vi "test_ccd_timerResolution.vi"(8 "error in":errorcluster, 11 "CCD in":refnum<class "CCD.lvclass">) -> (0 "error out":errorcluster, 3 "CCD out":refnum<class "CCD.lvclass">)   [LabVIEW 2023, in "horiba.test.lvlib"]
uses:
  horiba.test.lvlib
  Classes/CCD/CCD.lvclass
  C:/Projects/Horiba/horiba-labview-sdk/Source/Classes/GenericDevice/GenericDevice.lvclass
  15e7fe39-3d4f-4ccc-ae5c-22e5f2c5c50b.vi
  <vilib>/addons/_JKI Toolkits/Caraya/classes/Assert/Assert Equal Value and Type_Variant.vi
  <vilib>/addons/_JKI Toolkits/Caraya/classes/Test/Test.lvclass
  <vilib>/addons/_JKI Toolkits/Caraya/classes/Assert/Assert.lvclass
  <userlib>/_OpenG.lib/lvdata/lvdata.llb/openg_variant.lvlib
panel:
  # "Connector Pane"
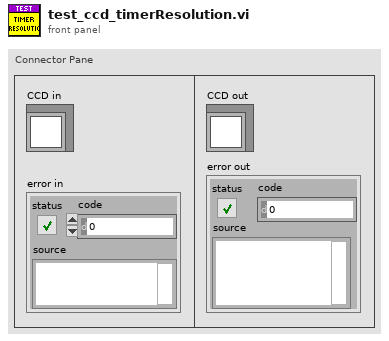
[diagram p1: front panel]
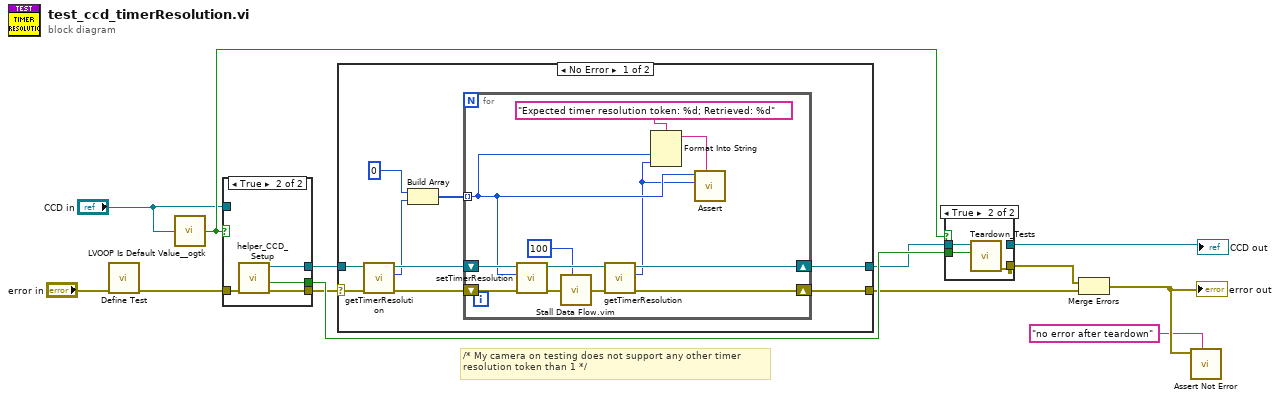
[diagram p0: block diagram]
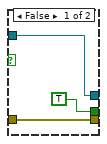
[diagram p3: hidden frame]
diagram:
  # "/* My camera on testing does not support any other timer \nresolution token than 1 */"
  n1 = call <vilib>:"Define Test.vi"("error in (no error)"="error in") -> ("error out"=w8:errorcluster)  [unwired: 9 in, 1 out]
  n2 = call <userlib>:"LVOOP Is Default Value__ogtk.vi"("Object"="CCD in") -> ("Is Default Value?"=w9:bool)
  n3 = case shown="True" w9 {
    tunnel: w8 -> [w15 w20]
    tunnel: [w15 w19] -> w4
    tunnel: [w16 w18] -> w6
    tunnel: [TRUE ("Module Was Already Running?") w17] -> w10
    tunnel: "CCD in" -> [w16 _]
    frame False {
    }
    frame True {
      n4 = call "helper_CCD_Setup.vi"("error in"=w20) -> ("error out"=w19:errorcluster, "Module Was Already Running?"=w17:bool, "CCD out"=w18:refnum<class "CCD.lvclass">)  [unwired: 7 in, 1 out]
    }
  }
  n5 = case shown="No Error" w4 {
    selector: w4 -> [w29 w42]
    tunnel: [w26 w43] -> w5
    tunnel: w6 -> [w28 w43]
    tunnel: [w24 w42] -> w3
    frame No Error {
      n6 = call "getTimerResolution.vi"("error in (no error)"=w29, "CCD in"=w28) -> ("error out"=w25:errorcluster, "resolutionToken"=w22:i32, "CCD out"=w27:refnum<class "CCD.lvclass">)  [unwired: 7 in]
      n7 = Build Array(0 ("token"), w22) -> (w21:i32[])
      n8 = for {
        shift-right: [w38] -> w26
        shift-left: w27 -> [w39]
        shift-right: [w36] -> w24
        shift-left: w25 -> [w37]
        tunnel: w21 -> [w33] mode=indexing
        n9 = call "setTimerResolution.vi"("error in (no error)"=w37, "resolutionToken"=w33, "CCD in"=w39) -> ("error out"=w41:errorcluster, "CCD out"=w40:refnum<class "CCD.lvclass">)  [unwired: 5 in, 2 out]
        n10 = call "Stall Data Flow.vim"("value in"=w41, "milliseconds to wait"=u32 100) -> ("value out"=w31:errorcluster)  [unwired: 1 out]
        n11 = call "getTimerResolution.vi"("error in (no error)"=w31, "CCD in"=w40) -> ("error out"=w36:errorcluster, "resolutionToken"=w32:i32, "CCD out"=w38:refnum<class "CCD.lvclass">)  [unwired: 7 in]
        n12 = Format Into String(format string="Expected timer resolution token: %d; Retrieved: %d", w33, w32) -> (resulting string=w35:string)  [unwired: 2 in, 1 out]
        n13 = call-poly <vilib>:"Assert.vi"("Label"=w35, "Y"=w32, "X"=w33) -> ()  [unwired: 7 in, 2 out]
      }
    }
    frame Error {
    }
  }
  n14 = case shown="True" w9 {
    tunnel: w5 -> [w44 w47]
    tunnel: [_ w46] -> w7
    tunnel: w10 -> [_ w45]
    tunnel: [w44 _] -> w1
    frame False {
    }
    frame True {
      n15 = call "Teardown_Tests.vi"("Module Was Already Running?"=w45, "horiba.lvlib:GenericDevice"=w47) -> ("error out"=w46:errorcluster)  [unwired: 8 in, 1 out]
    }
  }
  "CCD out" <- w1
  n16 = Merge Errors(w7, w3) -> (w12:errorcluster)
  "error out" <- w12
  n17 = call <vilib>:"Assert Not Error.vi"("Label"="no error after teardown", "Not Error?"=w12) -> ()  [unwired: 8 in, 2 out]
